vi "dvp Vi Set Config String.vi"(9 "pszValue":string, 10 "pszName":string, 11 "handle":u32) -> (1 "pszValue out":string, 2 "pszName out":string, 3 "function return":u32(ring))   [LabVIEW 2018, in "LabViewDVPCamera.lvlib"]
doc: "LabviewDvp2Api dvpStatus dvpViSetConfigString(dvpHandle handle,char *pszName,char *pszValue);"
uses:
  LabViewDVPCamera.lvlib
  LabViewDVPCamera/LabViewDVPCamera.dll
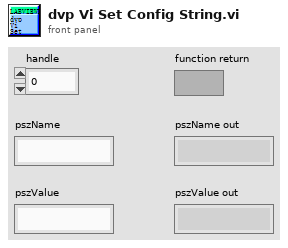
[diagram p1: front panel]
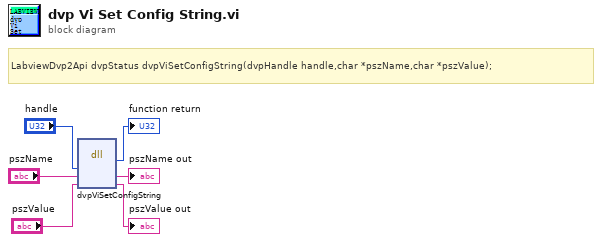
[diagram p0: block diagram]
diagram:
  # "LabviewDvp2Api dvpStatus dvpViSetConfigString(dvpHandle handle,char *pszName,char *pszValue);"
  n1 = dll-call lib="C:/Program Files (x86)/DVP2 Labview cn 64/Sample/LabViewDVPCamera/LabViewDVPCamera.*" fn="dvpViSetConfigString"("handle"="handle", "pszName"="pszName", "pszValue"="pszValue") -> (→"function return":u32, "pszName"=→"pszName out":string, "pszValue"=→"pszValue out":string)  [unwired: 4 in, 2 out]
